vi "Credentials Error Interception.vi"(8 "error in":errorcluster, 11 "Target settings in":T1 {"Primary NIC"."IP Address Request Mode" items=["Static"=1, "DHCP/Link-Local"=2, "Link-Local Only"=4, "DHCP Only"=8]}) -> (0 "error out":errorcluster, 3 "Target settings out":T1 {"Primary NIC"."IP Address Request Mode" items=["Static"=1, "DHCP/Link-Local"=2, "Link-Local Only"=4, "DHCP Only"=8]})   [LabVIEW 2020]
uses:
  SubVIs/Target Information.ctl
  subVIs/Targets/TypeDefs/rad_Target Network Settings.ctl
  SubVIs/System Credentials.ctl
  <vilib>/nisyscfg/Close (System).vi
  <vilib>/nisyscfg/nisyscfg.lvlib
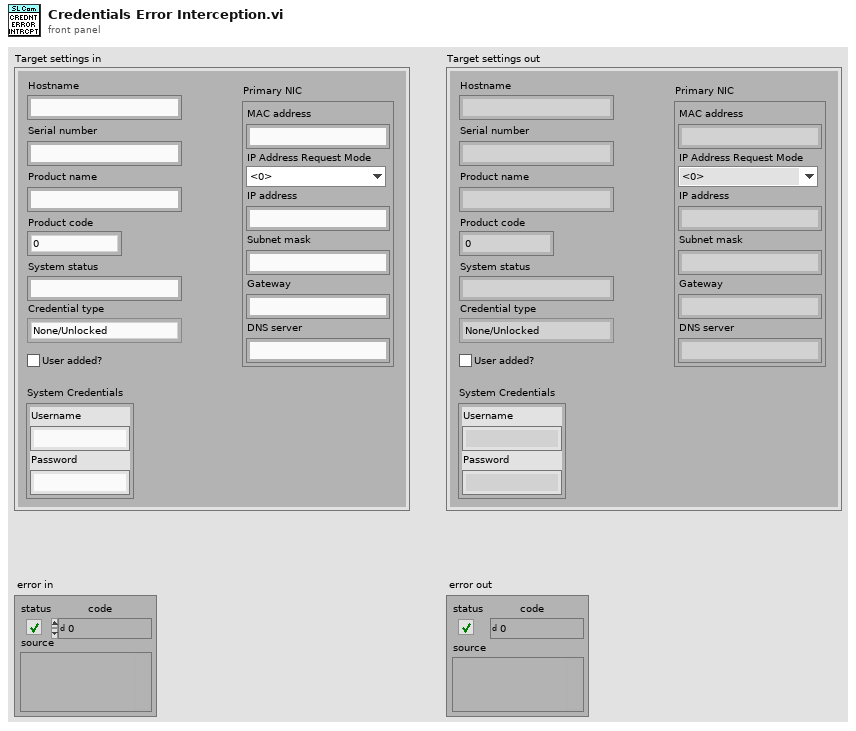
[diagram p1: front panel]
types:
  T1 = typedef "Target Information.ctl" = cluster{"Hostname":string, "Serial number":string, "Product name":string, "Product code":i32, "System status":string, "Credential type":enum16{"None/Unlocked", "FTP Password", "NIAuth Credentials"}, "User added?":bool, "Primary NIC":T2, "System Credentials":T3}
  T2 = typedef "rad_Target Network Settings.ctl" = cluster{"MAC address":string, "IP Address Request Mode":i32, "IP address":string, "Subnet mask":string, "Gateway":string, "DNS server":string}
  T3 = typedef "System Credentials.ctl" = cluster{"Username":string, "Password":string}
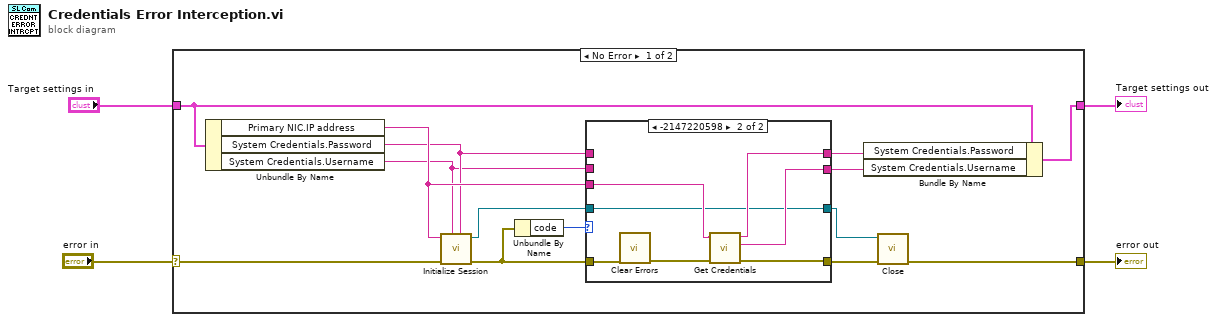
[diagram p0: block diagram]
diagram:
  n1 = case shown="No Error" "error in" {
    selector: "error in" -> [w18 w31]
    tunnel: "Target settings in" -> [w7 w30]
    tunnel: [w14 w31] -> w2
    tunnel: [w8 w30] -> w1
    frame No Error {
      n2 = Unbundle By Name(w7) -> ("Primary NIC.IP address"=w13:string, "System Credentials.Password"=w10:string, "System Credentials.Username"=w5:string)
      n3 = call <vilib>:"Initialize Session.vi"("Password"=w10, "User Name"=w5, "error in (no error)"=w18, "Target (localhost)"=w13) -> ("error out"=w16:errorcluster, "Session out"=w12:refnum<k21>)  [unwired: 6 in]
      n4 = Unbundle By Name(w16) -> ("code"=w17:i32)
      n5 = case shown="-2147220598" w17 {
        tunnel: [w22 w26] -> w15
        tunnel: w16 -> [w22 w29]
        tunnel: [w21 w25] -> w9
        tunnel: w10 -> [w21 _]
        tunnel: [w19 w24] -> w6
        tunnel: w13 -> [_ w27]
        tunnel: w12 -> [w20 w23]
        tunnel: [w20 w23] -> w11
        tunnel: w5 -> [w19 _]
        frame 0, Default {
        }
        frame -2147220598 {
          n6 = call <vilib>:"Clear Errors.vi"("error in (no error)"=w29) -> ("error out"=w28:errorcluster)  [unwired: 5 in, 1 out]
          n7 = call "Get Credentials.vi"("error in"=w28, "IP Address"=w27) -> ("error out"=w26:errorcluster, "Password"=w24:string, "User name"=w25:string)  [unwired: 7 in]
        }
      }
      n8 = Bundle By Name(cluster=w7, "System Credentials.Password"=w9, "System Credentials.Username"=w6) -> (w8:T1)
      n9 = call-poly <vilib>:"Close.vi"("error in (no error)"=w15, "Session in"=w11) -> ("error out"=w14:errorcluster)  [unwired: 9 in]
    }
    frame Error {
    }
  }
  "error out" <- w2
  "Target settings out" <- w1
